vi "Log Rectifier Settings.vi"(4 "Amp-min Left Anode":dbl, 6 "Right Anode Output":dbl, 7 "Panel Name":string, 8 "error in (no error)":errorcluster, 9 "Left Anode Output":dbl, 10 "Amp-min Right Anode":dbl, 11 "Tank Number":string) -> (0 "error out":errorcluster)   [LabVIEW 2019]
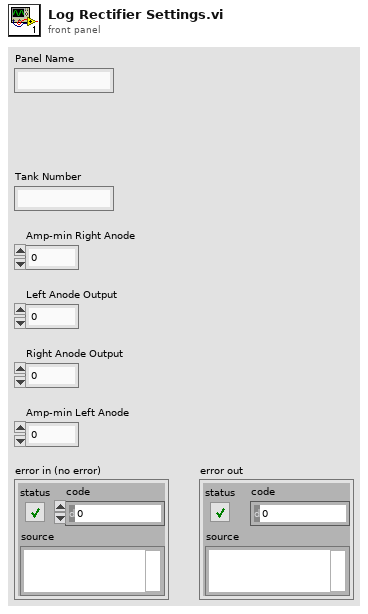
[diagram p1: front panel]
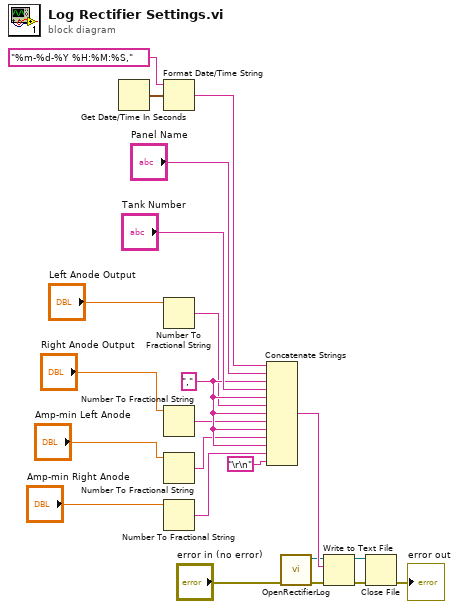
[diagram p0: block diagram]
diagram:
  w13 = "," ("string")
  n1 = Get Date/Time In Seconds() -> (seconds since 1Jan1904=w1:timestamp)
  n2 = Format Date/Time String(time format string (%c)="%m-%d-%Y %H:%M:%S,", seconds (now)=w1) -> (date/time string=w3:string)  [unwired: 1 in]
  n3 = Number To Fractional String(number="Left Anode Output") -> (F-format string=w6:string)  [unwired: 3 in]
  n4 = Number To Fractional String(number="Right Anode Output") -> (F-format string=w8:string)  [unwired: 3 in]
  n5 = Number To Fractional String(number="Amp-min Left Anode") -> (F-format string=w11:string)  [unwired: 3 in]
  n6 = Number To Fractional String(number="Amp-min Right Anode") -> (F-format string=w12:string)  [unwired: 3 in]
  n7 = Concatenate Strings(w3, "Panel Name", w13, "Tank Number", w13, w6, w13, w8, w13, w11, w13, w12, "\r\n") -> (w15:string)
  n8 = call "OpenRectifierLog.vi"("error in (no error)"="error in (no error)") -> ("error out"=w16:errorcluster, "Fileref out"=w14:refnum<file>)  [unwired: 9 in]
  n9 = Write to Text File(file (use dialog)=w14, text=w15, error in=w16) -> (refnum out=w17:refnum<file>, error out=w18:errorcluster)  [unwired: 1 in, 1 out]
  n10 = Close File(refnum=w17, error in=w18) -> (error out=→"error out":errorcluster)  [unwired: 1 out]
